vi "Read(I32).vi"(8 "错误输入":errorcluster, 11 "TagName":string) -> (0 "错误输出":errorcluster, 3 "Data":sgl)   [LabVIEW 2013, in "Tag Data by Variant.lvlib"]
uses:
  Tag Data by Variant.lvlib
  Custom def/mode.ctl
  Core/TagVar Data(I32).vi
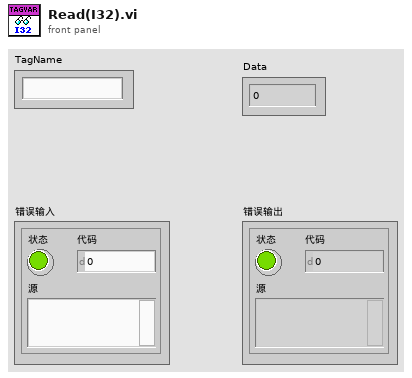
[diagram p1: front panel]
types:
  T1 = typedef "Tag Data by Variant.lvlib/mode.ctl" = enum16{"初始化", "加入", "删除", "读取", "读取所有", "清除"}
  T2 = typedef "Tag Data by Variant.lvlib/Tag I32.ctl" = cluster{"Name":string, "Data":i32}
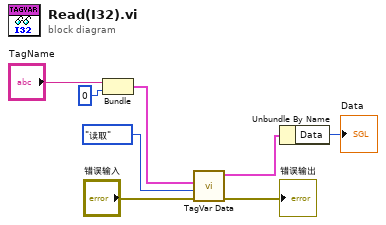
[diagram p0: block diagram]
diagram:
  n1 = Bundle("TagName"="TagName", 0) -> (w3:cluster{"TagName":string, i32})  [unwired: 1 in]
  n2 = call-poly "TagVar Data.vi"("错误输入"="错误输入", "method"=mode."读取", "TagData"=w3) -> ("错误输出"=→"错误输出":errorcluster, "TagData"=w2:T2)  [unwired: 6 in, 1 out]
  n3 = Unbundle By Name(w2) -> ("Data"=→"Data":i32)
